vi "write_params.vi"(8 "error in (no error)":errorcluster caption="entrée d'erreur (pas d'erreur)", 10 "params":T1={"loss"="hinge", "penalty"="l2", "alpha"=0.001, "l1_ratio"=0.15, "fit_intercept"=TRUE, "max_iter"=1000.0, "tol"=0.001, "shuffle"=TRUE, "n_jobs"=1.0, "random_state"=0.0, "learning_rate"="optimal", "eta0"=0.0, "power_t"=0.5, "early_stopping"=FALSE, "validation_fraction"=0.1, "n_iter_no_change"=5.0, "class_weight"={"class_weight_type"="None", "class_weight_dict"="{\"class_label\":1.2}"}, "warm_start"=FALSE, "average"={"average_type"="bool", "average_bool"=FALSE, "average_int"=0.0}}, 11 "SGDClassifier en entrée":refnum<class "SGDClassifier.lvclass">) -> (0 "error out":errorcluster caption="sortie d'erreur", 3 "SGDClassifier en sortie":refnum<class "SGDClassifier.lvclass">)   [LabVIEW 2020, in "SGDClassifier.lvclass"]
uses:
  SGDClassifier.lvclass
  Controls/sgdclassifier_params.ctl
  SGDClassifier.lvclass/SGDClassifier.ctl
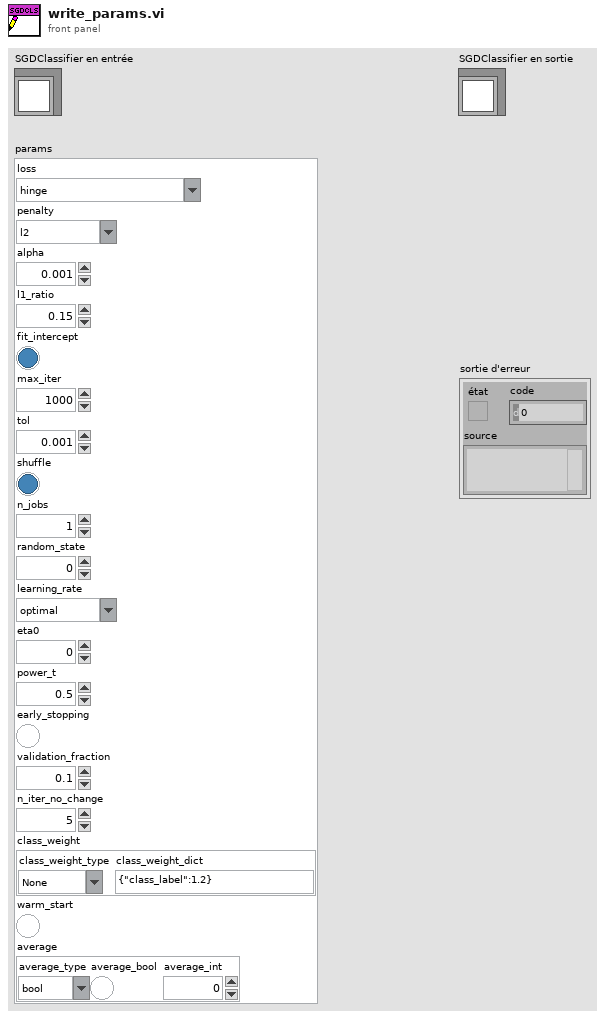
[diagram p1: front panel]
types:
  T1 = typedef "sgdclassifier_params.ctl" = cluster{"loss":string, "penalty":string, "alpha":dbl, "l1_ratio":dbl, "fit_intercept":bool, "max_iter":dbl, "tol":dbl, "shuffle":bool, "n_jobs":dbl, "random_state":dbl, "learning_rate":string, "eta0":dbl, "power_t":dbl, "early_stopping":bool, "validation_fraction":dbl, "n_iter_no_change":dbl, "class_weight":cluster{"class_weight_type":string, "class_weight_dict":string}, "warm_start":bool, "average":cluster{"average_type":string, "average_bool":bool, "average_int":dbl}}
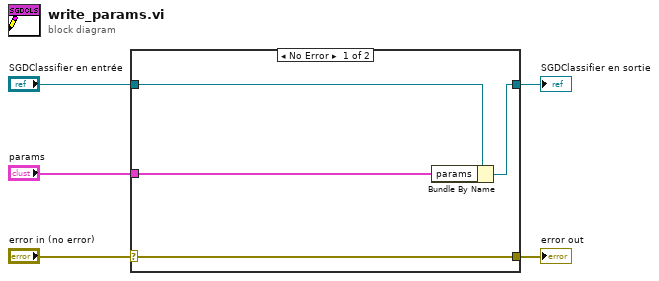
[diagram p0: block diagram]
diagram:
  n1 = case shown="No Error" "error in (no error)" {
    selector: "error in (no error)" -> [w9 w10]
    tunnel: [w9 w10] -> w4
    tunnel: [w7 w11] -> w2
    tunnel: "SGDClassifier en entrée" -> [w8 w11]
    tunnel: "params" -> [w6 _]
    frame No Error {
      n2 = Bundle By Name(cluster=w8, "params"=w6) -> (w7:refnum<class "SGDClassifier.lvclass">)
    }
    frame Error {
    }
  }
  "error out" <- w4
  "SGDClassifier en sortie" <- w2
